vi "Sample--Sync_ExtClk_USB.vi"() -> ()   [LabVIEW 2013]
doc: "This example demonstrates synchronizing two digitizers."
uses:
  <userlib>/ArtScope/Trigger/ArtScope_ConfigureTriggerDigital.vi
  <userlib>/ArtScope/Fetch/ArtScope_FetchBinary16.vi
  <userlib>/ArtScope/_SubVI/ArtScope_ArrayByChannel_U16.vi
panel:
  in  "reference position2":dbl
  in  "reference position":dbl
  in  "range(Vpp) 2":i32(ring) items=["20V", "10V", "2V", "40V", "16V", "8V", "4V", "1.6V", "800m", "400m", "160m", "80m", "40m"]
  in  "range(Vpp)":i32(ring) items=["20V", "10V", "2V", "40V", "16V", "8V", "4V", "1.6V", "800m", "400m", "160m", "80m", "40m"]
  in  "Slave":string="Dev2"
  in  "Master":string="Dev1"
  in  "Stop":bool
  out "Data2":u16[][](graph)
  in  "Timeout(s) 2":dbl=1.0
  in  "MinSampleRate 2":dbl=8000000.0
  in  "MinRecordLength2":i32=6000
  out "Data":u16[][](graph)
  out "ErrorOutput":errorcluster
  in  "Timeout(s)":dbl=1.0
  in  "MinRecordLength":i32=6000
  in  "MinSampleRate":dbl=8000000.0
  # "Vertical"
  # "Horizontal"
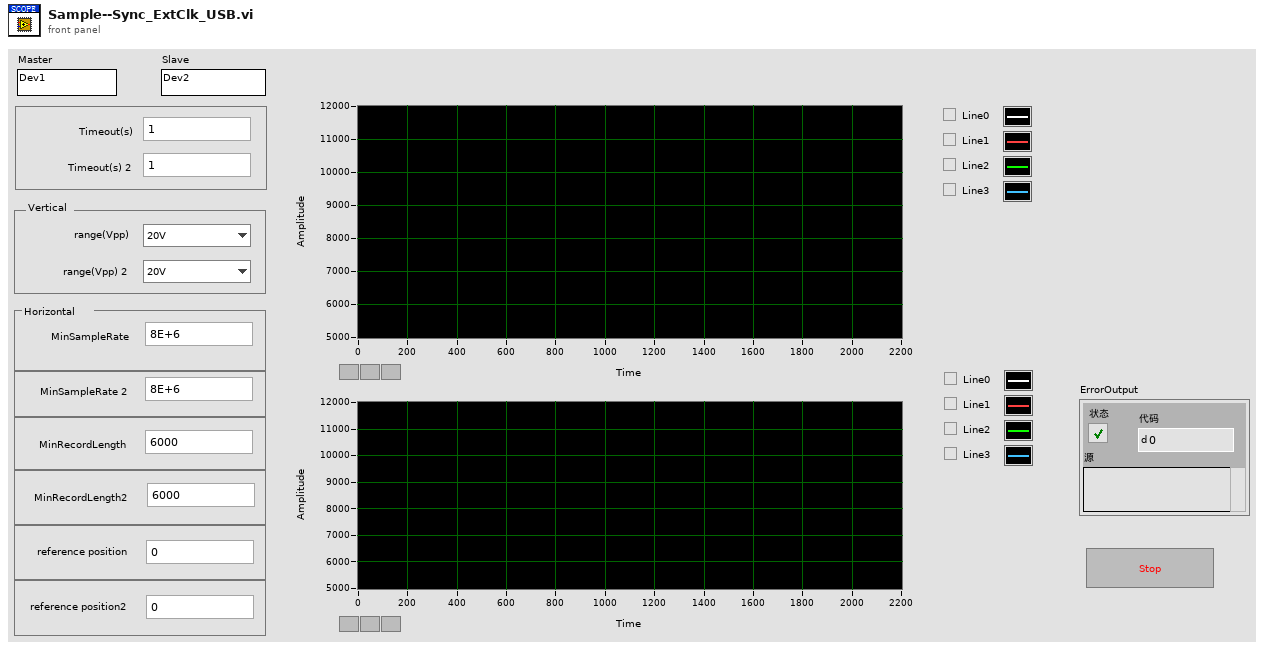
[diagram p1: front panel]
types:
  T1 = cluster{"fLSB":cluster{dbl, dbl, dbl, dbl, dbl, dbl, dbl, dbl}, "RangeValue":cluster{dbl, dbl, dbl, dbl, dbl, dbl, dbl, dbl}, "wMaxLSB":u32, "TriggerMode":i32, "sampLengthPerChan":u32, "pAvailSampsPoints":u32, "channelCount":i32}
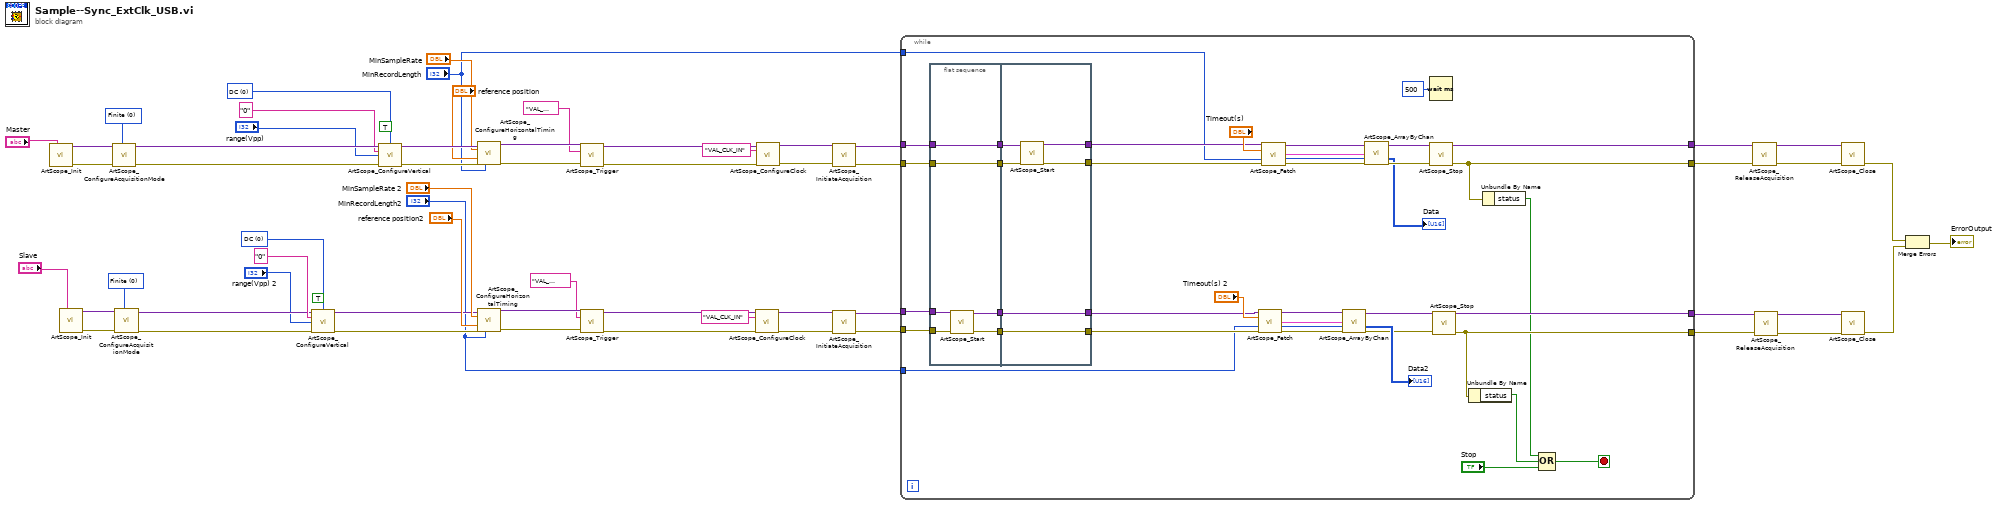
[diagram p0: block diagram]
diagram:
  (unwired) TRUE ("Enable")
  (unwired) TRUE ("Enable")
  w38 = 0 items=["DC", "AC"] ("Coupling")
  w46 = 0 items=["Finite", "Continuous"] ("AcuqMode")
  w56 = 0 items=["DC", "AC"] ("Coupling")
  w51 = 0 items=["Finite", "Continuous"] ("AcuqMode")
  n1 = call <userlib>:"ArtScope_Init.vi"("task name"="Master") -> ("task handle"=w33:variant, "error out"=w32:errorcluster)  [unwired: 13 in]
  n2 = call <userlib>:"ArtScope_Init.vi"("task name"="Slave") -> ("task handle"=w30:variant, "error out"=w29:errorcluster)  [unwired: 13 in]
  n3 = call <userlib>:"ArtScope_ConfigureAcquisitionMode.vi"("task handle"=w33, "acquisition mode"=w51, "error in (no error)"=w32) -> ("task handle"=w50:variant, "error out"=w52:errorcluster)  [unwired: 11 in]
  n4 = call <userlib>:"ArtScope_ConfigureAcquisitionMode.vi"("task handle"=w30, "acquisition mode"=w46, "error in (no error)"=w29) -> ("task handle"=w37:variant, "error out"=w36:errorcluster)  [unwired: 11 in]
  n5 = call <userlib>:"ArtScope_ConfigureVertical.vi"("task handle"=w37, "coupling"=w38, "channels"="0" ("Channel Name"), "range(Vpp)"="range(Vpp) 2", "error in (no error)"=w36) -> ("task handle"=w39:variant, "error out"=w40:errorcluster)  [unwired: 9 in]
  n6 = call <userlib>:"ArtScope_ConfigureVertical.vi"("task handle"=w50, "coupling"=w56, "channels"="0" ("Channel Name"), "range(Vpp)"="range(Vpp)", "error in (no error)"=w52) -> ("task handle"=w55:variant, "error out"=w54:errorcluster)  [unwired: 9 in]
  n7 = call <userlib>:"ArtScope_ConfigureHorizontalTiming.vi"("task handle"=w55, "min sample rate"="MinSampleRate", "reference position"="reference position", "error in (no error)"=w54, "min record length"="MinRecordLength") -> ("task handle"=w35:variant, "error out"=w49:errorcluster)  [unwired: 9 in]
  n8 = call <userlib>:"ArtScope_ConfigureHorizontalTiming.vi"("task handle"=w39, "min sample rate"="MinSampleRate 2", "reference position"="reference position2", "error in (no error)"=w40, "min record length"="MinRecordLength2") -> ("task handle"=w43:variant, "error out"=w42:errorcluster)  [unwired: 9 in]
  n9 = call-poly <userlib>:"ArtScope_Trigger.vi"("task handle"=w35, "trigger source"="VAL_TRIGGER_DTR", "error in"=w49) -> ("task handle"=w6:variant, "error out"=w5:errorcluster)  [unwired: 11 in]
  n10 = call-poly <userlib>:"ArtScope_Trigger.vi"("task handle"=w43, "trigger source"="VAL_TRIGGER_SYNCTRIGGER" ("TriggerSource"), "error in"=w42) -> ("task handle"=w4:variant, "error out"=w3:errorcluster)  [unwired: 11 in]
  n11 = call <userlib>:"ArtScope_ConfigureClock.vi"("task handle"=w4, "input clock source"="VAL_CLK_IN", "error in (no error)"=w3) -> ("task handle"=w27:variant, "error out"=w25:errorcluster)  [unwired: 11 in]
  n12 = call <userlib>:"ArtScope_ConfigureClock.vi"("task handle"=w6, "input clock source"="VAL_CLK_IN", "error in (no error)"=w5) -> ("task handle"=w21:variant, "error out"=w23:errorcluster)  [unwired: 11 in]
  n13 = call <userlib>:"ArtScope_InitiateAcquisition.vi"("task handle"=w27, "error in (no error)"=w25) -> ("task handle"=w26:variant, "error out"=w24:errorcluster)  [unwired: 12 in]
  n14 = call <userlib>:"ArtScope_InitiateAcquisition.vi"("task handle"=w21, "error in (no error)"=w23) -> ("task handle"=w20:variant, "error out"=w22:errorcluster)  [unwired: 12 in]
  n15 = while {
    tunnel: [w96] -> w19
    tunnel: [w83] -> w17
    tunnel: [w85] -> w15
    tunnel: [w95] -> w12
    tunnel: w26 -> [w94]
    tunnel: w24 -> [w93]
    tunnel: w20 -> [w89]
    tunnel: w22 -> [w88]
    tunnel: "MinRecordLength" -> [w75]
    tunnel: "MinRecordLength2" -> [w74]
    stop <- w80 stop-if-true
    n16 = flat-sequence {
      tunnel: w94 -> [w104]
      tunnel: w93 -> [w103]
      tunnel: [w99] -> w98
      tunnel: [w102] -> w97
      tunnel: [w101] -> w90
      tunnel: w89 -> [w101]
      tunnel: w88 -> [w100]
      tunnel: [w100] -> w87
      tunnel: w98 -> [w110]
      tunnel: w97 -> [w109]
      tunnel: w90 -> [w108]
      tunnel: w87 -> [w107]
      tunnel: [w110] -> w79
      tunnel: [w109] -> w78
      tunnel: [w106] -> w77
      tunnel: [w105] -> w76
      frame #0 {
        n17 = call <userlib>:"ArtScope_Start.vi"("task handle"=w104, "error in (no error)"=w103) -> ("task handle"=w99:variant, "error out"=w102:errorcluster)  [unwired: 12 in]
      }
      frame #1 {
        n18 = call <userlib>:"ArtScope_Start.vi"("task handle"=w108, "error in (no error)"=w107) -> ("task handle"=w106:variant, "error out"=w105:errorcluster)  [unwired: 12 in]
      }
    }
    n19 = call-poly <userlib>:"ArtScope_Fetch.vi"("task handle"=w79, "timeout"="Timeout(s) 2", "num samples"=w74, "error in (no error)"=w78) -> ("task handle"=w63:variant, "wfm info"=w61:T1, "data"=w60:u16[], "error out"=w62:errorcluster)  [unwired: 8 in]
    n20 = call-poly <userlib>:"ArtScope_Fetch.vi"("task handle"=w77, "timeout"="Timeout(s)", "num samples"=w75, "error in (no error)"=w76) -> ("task handle"=w73:variant, "wfm info"=w68:T1, "data"=w67:u16[], "error out"=w72:errorcluster)  [unwired: 8 in]
    n21 = call-poly <userlib>:"ArtScope_ArrayByChan.vi"("task handle"=w63, "wfm info"=w61, "1D data"=w60, "error in (no error)"=w62) -> ("task handle"=w64:variant, "2D data"=→"Data2":u16[][], "error out"=w65:errorcluster)  [unwired: 9 in]
    n22 = call-poly <userlib>:"ArtScope_ArrayByChan.vi"("task handle"=w73, "wfm info"=w68, "1D data"=w67, "error in (no error)"=w72) -> ("task handle"=w70:variant, "2D data"=→"Data":u16[][], "error out"=w71:errorcluster)  [unwired: 9 in]
    n23 = call <userlib>:"ArtScope_Stop.vi"("task handle"=w70, "error in"=w71) -> ("task handle"=w96:variant, "error out"=w83:errorcluster)  [unwired: 12 in]
    n24 = Wait (ms)(milliseconds to wait=u32 500 ("等待时间（毫秒）")) -> ()  [unwired: 1 out]
    n25 = call <userlib>:"ArtScope_Stop.vi"("task handle"=w64, "error in"=w65) -> ("task handle"=w95:variant, "error out"=w85:errorcluster)  [unwired: 12 in]
    n26 = Unbundle By Name(w85) -> ("status"=w84:bool)
    n27 = Unbundle By Name(w83) -> ("status"=w82:bool)
    n28 = Compound Arithmetic op=OR(w82, w84, "Stop") -> (w80:bool)
  }
  n29 = call <userlib>:"ArtScope_ReleaseAcquisition.vi"("task handle"=w19, "error in (no error)"=w17) -> ("task handle"=w18:variant, "error out"=w16:errorcluster)  [unwired: 12 in]
  n30 = call <userlib>:"ArtScope_ReleaseAcquisition.vi"("task handle"=w12, "error in (no error)"=w15) -> ("task handle"=w13:variant, "error out"=w14:errorcluster)  [unwired: 12 in]
  n31 = call <userlib>:"ArtScope_Close.vi"("task handle"=w18, "error in (no error)"=w16) -> ("error out"=w59:errorcluster)  [unwired: 13 in]
  n32 = call <userlib>:"ArtScope_Close.vi"("task handle"=w13, "error in (no error)"=w14) -> ("error out"=w58:errorcluster)  [unwired: 13 in]
  n33 = Merge Errors(w59, w58) -> (→"ErrorOutput":errorcluster)
